vi "Read mecury field RS232.vi"(8 "error in (no error)":errorcluster, 10 "Device on PSU":string, 11 "VISA resource name":refnum<visa-resource-name>) -> (0 "error out":errorcluster, 2 "FIeld mT":dbl, 3 "VISA resource name out":refnum<visa-resource-name>)   [LabVIEW 2024]
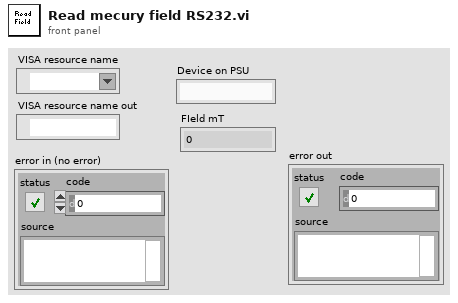
[diagram p1: front panel]
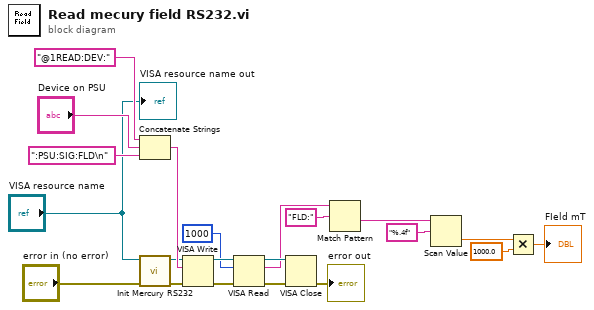
[diagram p0: block diagram]
diagram:
  n1 = Concatenate Strings("@1READ:DEV:" ("string"), "Device on PSU", ":PSU:SIG:FLD\n" ("string")) -> (w18:string)
  n2 = call "Init Mercury RS232.vi"("error in (no error)"="error in (no error)", "VISA resource name"="VISA resource name") -> ("error out"=w9:errorcluster, "VISA resource name out"=w8:refnum<visa-resource-name>)  [unwired: 8 in]
  n3 = VISA Write(VISA resource name=w8, write buffer=w18, error in (no error)=w9) -> (VISA resource name out=w17:refnum<visa-resource-name>, error out=w16:errorcluster)  [unwired: 1 out]
  n4 = VISA Read(VISA resource name=w17, byte count=u32 1000, error in (no error)=w16) -> (VISA resource name out=w5:refnum<visa-resource-name>, read buffer=w3:string, error out=w7:errorcluster)  [unwired: 1 out]
  n5 = VISA Close(VISA resource name=w5, error in (no error)=w7) -> (error out=→"error out":errorcluster)
  n6 = Match Pattern(string=w3, regular expression="FLD:") -> (after substring=w1:string)  [unwired: 1 in, 3 out]
  n7 = Scan Value(string=w1, format string="%.4f") -> (value=w13:dbl)  [unwired: 1 in, 1 out]
  n8 = Multiply(x=w13, y=1000.0) -> (x*y=→"FIeld mT":dbl)
  "VISA resource name out" <- "VISA resource name"
